vi "_loop_time.vi"(11 "from shift register":dbl) -> (2 "loop time (ms)":dbl, 3 "to shift register":dbl)   [LabVIEW 2024]
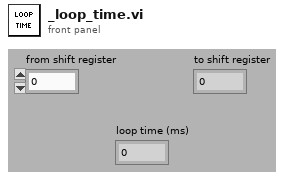
[diagram p1: front panel]
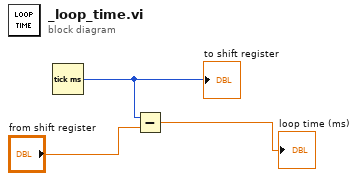
[diagram p0: block diagram]
diagram:
  n1 = Tick Count (ms)() -> (millisecond timer value=w2:u32)
  "to shift register" <- w2
  n2 = Subtract(x=w2, y="from shift register") -> (x-y=→"loop time (ms)":dbl)
